vi "Disconnect.vi"(8 "error in (no error)":errorcluster, 11 "Omega CN9600 series.lvclass":refnum<class "Omega CN9600 series.lvclass">) -> (0 "error out":errorcluster)   [LabVIEW 2014, in "Omega CN9600 series.lvclass"]
uses:
  Omega CN9600 series.lvclass
  Omega CN9600 series.lvclass/Omega CN9600 series.ctl
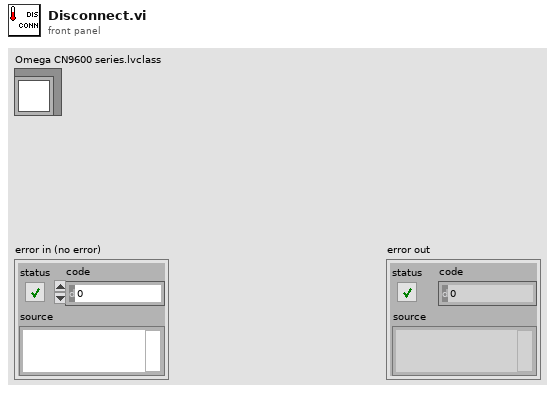
[diagram p1: front panel]
types:
  T1 = typedef "Omega CN9600 series.lvclass/Serial_Config_Omega.ctl" = cluster{"Baud":u32, "Flow Ctl":u16, "Parity":u16, "Address":u8, "VISA resource name":refnum<visa-resource-name>}
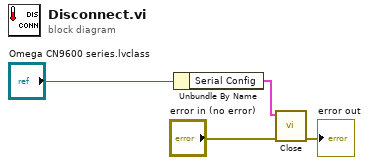
[diagram p0: block diagram]
diagram:
  n1 = Unbundle By Name("Omega CN9600 series.lvclass") -> ("Serial Config"=w1:T1)
  n2 = call "Close.vi"("error in (no error)"="error in (no error)", "Serial Config"=w1) -> ("error out"=→"error out":errorcluster)  [unwired: 9 in]
